vi "external cmd - parse string.vi"(0 "input cmd":string) -> (4 "address":u8, 6 "content":string, 8 "is true":bool, 10 "command ok":bool)   [LabVIEW 2010]
uses:
  <vilib>/Utility/error.llb/whitespace.ctl
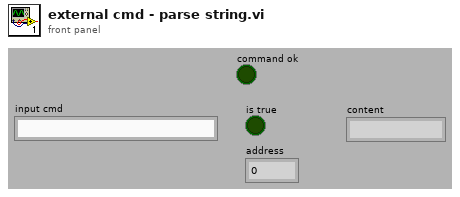
[diagram p1: front panel]
types:
  T1 = typedef "whitespace.ctl" = u16
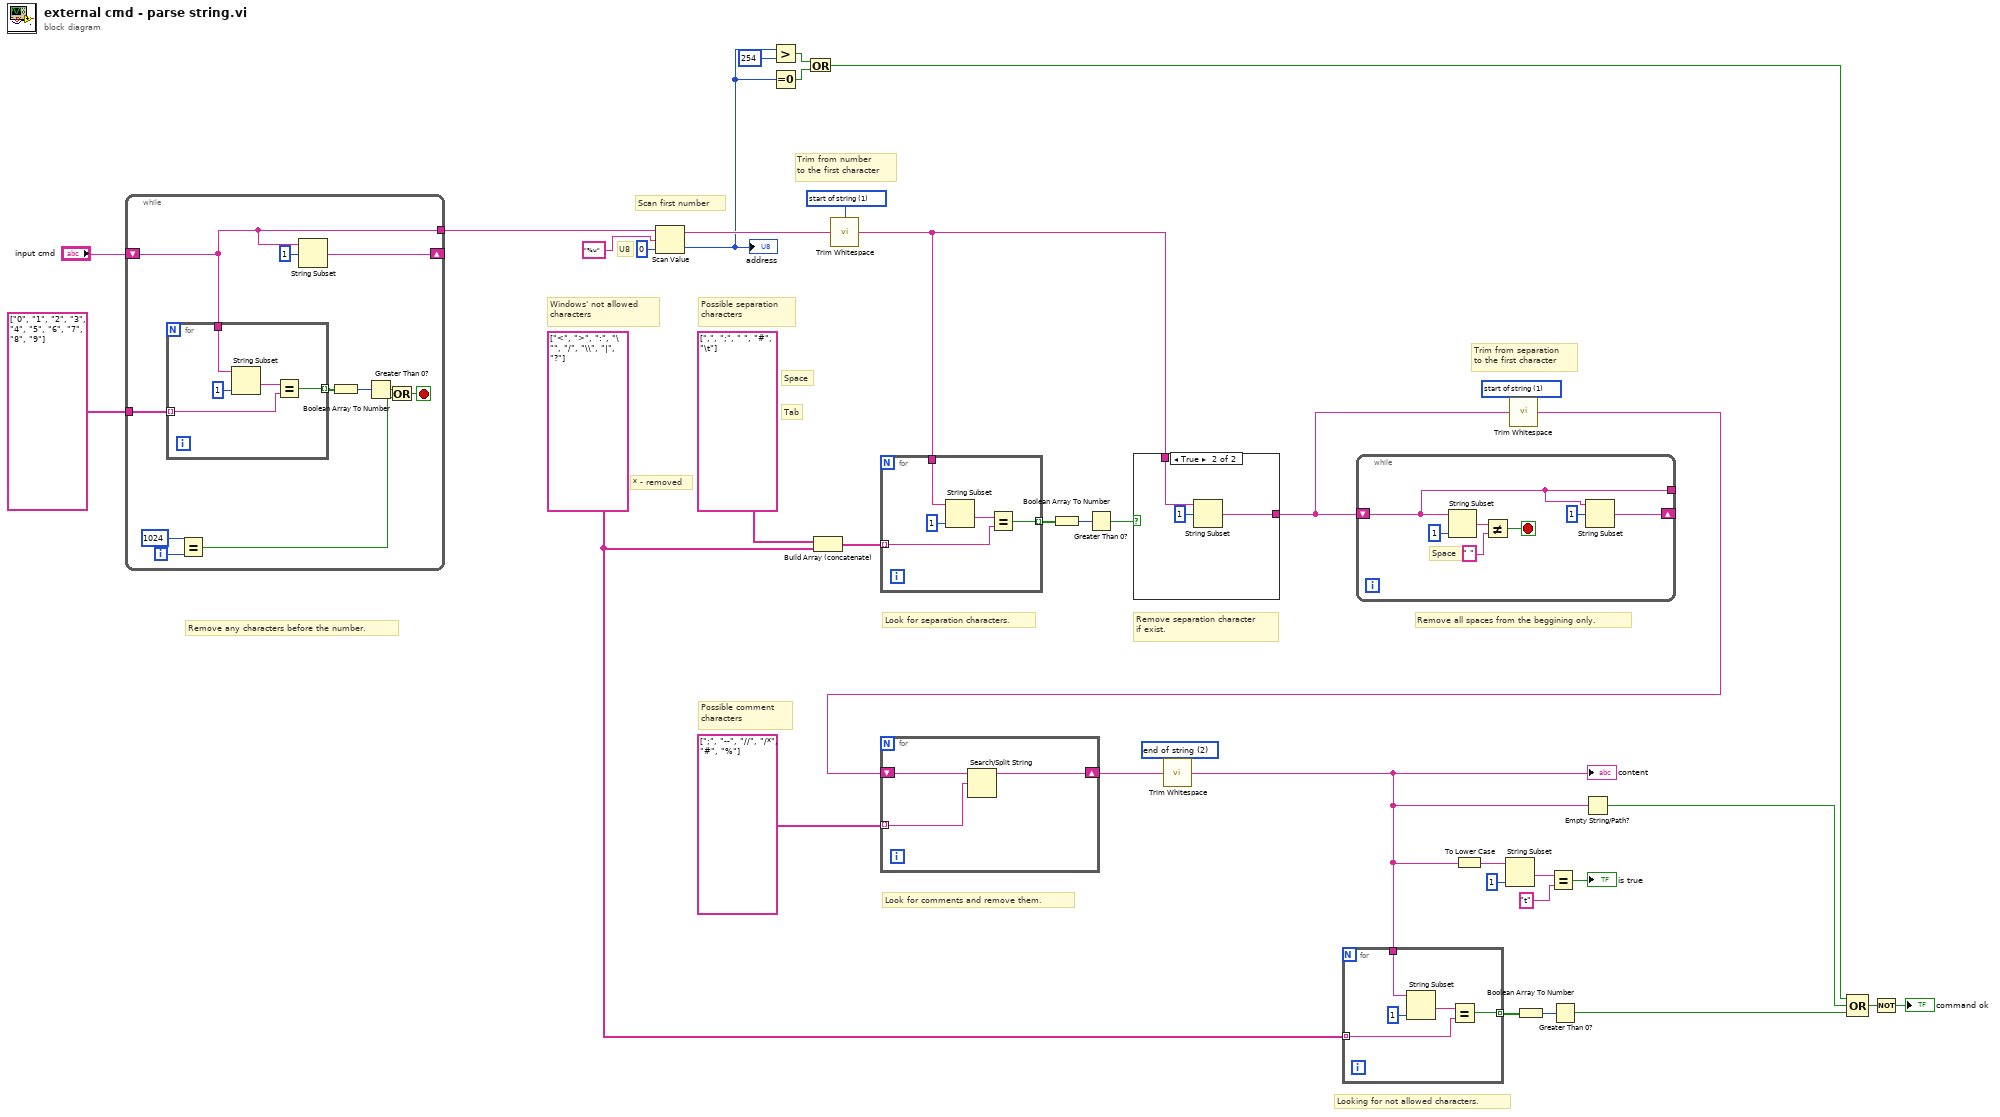
[diagram p0: block diagram]
diagram:
  w19 = T1 1 items=["both", "start of string", "end of string"] ("location (both)")
  w21 = T1 2 items=["both", "start of string", "end of string"] ("location (both)")
  w24 = T1 1 items=["both", "start of string", "end of string"] ("location (both)")
  w18 = string[] ["<", ">", ":", "\"", "/", "\\", "|", "?"]
  # "* - removed"
  # "Looking for not allowed characters."
  # "Trim from separation\nto the first character"
  # "Trim from number\nto the first character"
  # "Scan first number"
  # "Look for comments and remove them."
  # "Possible comment\ncharacters"
  # "Remove all spaces from the beggining only."
  # "Remove separation character\nif exist."
  # "Look for separation characters."
  # "Remove any characters before the number."
  # "Tab"
  # "Space"
  # "U8"
  # "Possible separation\ncharacters"
  # "Windows' not allowed\ncharacters"
  n1 = while {
    shift-right: [w47] -> _
    shift-left: "input cmd" -> [w42]
    tunnel: [w42] -> w28
    tunnel: string[] ["0", "1", "2", "3", "4", "5", "6", "7", "8", "9"] -> [w46]
    i -> [w41]
    stop <- w39 stop-if-true
    n2 = for {
      tunnel: w46 -> [w50] mode=indexing
      tunnel: w42 -> [w53]
      tunnel: [w49] -> w44 mode=indexing
      n3 = String Subset(string=w53, length (rest)=1 ("length (rest)")) -> (substring=w51:string)  [unwired: 1 in]
      n4 = Equal?(x=w51, y=w50) -> (x = y?=w49:bool)
    }
    n5 = Equal?(x=1024, y=w41) -> (x = y?=w38:bool)
    n6 = String Subset(string=w42, offset (0)=1) -> (substring=w47:string)  [unwired: 1 in]
    n7 = Boolean Array To Number(Boolean array=w44) -> (number=w45:u32)
    n8 = Greater Than 0?(x=w45) -> (x > 0?=w43:bool)
    n9 = Or(x=w43, y=w38) -> (x .or. y?=w39:bool)
  }
  n10 = Scan Value(string=w28, format string="%u", default (0 dbl)=u8 0) -> (output string=w25:string, value=w11:u8)
  "address" <- w11
  n11 = Greater?(x=w11, y=u8 254) -> (0:w9:bool)
  n12 = Equal To 0?(x=w11) -> (x = 0?=w10:bool)
  n13 = Or(x=w9, y=w10) -> (x .or. y?=w8:bool)
  n14 = Build Array (concatenate)(string[] [",", ";", " ", "#", "\t"], w18) -> (w35:string[])
  n15 = call <vilib>:"Trim Whitespace.vi"("string"=w25, "location (both)"=w19) -> ("trimmed string"=w20:string)
  n16 = for {
    tunnel: w35 -> [w55] mode=indexing
    tunnel: w20 -> [w58]
    tunnel: [w54] -> w33 mode=indexing
    n17 = String Subset(string=w58, length (rest)=1 ("length (rest)")) -> (substring=w56:string)  [unwired: 1 in]
    n18 = Equal?(x=w56, y=w55) -> (x = y?=w54:bool)
  }
  n19 = Boolean Array To Number(Boolean array=w33) -> (number=w32:u32)
  n20 = Greater Than 0?(x=w32) -> (x > 0?=w31:bool)
  n21 = case shown="True" w31 {
    tunnel: w20 -> [w59 w62]
    tunnel: [w59 w60] -> w23
    frame False {
    }
    frame True {
      n22 = String Subset(string=w62, offset (0)=1) -> (substring=w60:string)  [unwired: 1 in]
    }
  }
  n23 = while {
    shift-right: [w64] -> _
    shift-left: w23 -> [w63]
    tunnel: [w63] -> _
    stop <- w67 stop-if-true
    # "Space"
    n24 = String Subset(string=w63, length (rest)=1 ("length (rest)")) -> (substring=w65:string)  [unwired: 1 in]
    n25 = Not Equal?(x=w65, y=" " ("search string")) -> (x != y?=w67:bool)
    n26 = String Subset(string=w63, offset (0)=1) -> (substring=w64:string)  [unwired: 1 in]
  }
  n27 = call <vilib>:"Trim Whitespace.vi"("string"=w23, "location (both)"=w24) -> ("trimmed string"=w22:string)
  n28 = for {
    tunnel: string[] [";", "--", "//", "/*", "#", "%"] -> [w71] mode=indexing
    shift-right: [w70] -> w26
    shift-left: w22 -> [w72]
    n29 = Search/Split String(string=w72, search string/char (-)=w71) -> (substring before match=w70:string)  [unwired: 1 in, 2 out]
  }
  n30 = call <vilib>:"Trim Whitespace.vi"("string"=w26, "location (both)"=w21) -> ("trimmed string"=w14:string)
  "content" <- w14
  n31 = for {
    tunnel: w18 -> [w74] mode=indexing
    tunnel: w14 -> [w77]
    tunnel: [w73] -> w16 mode=indexing
    n32 = String Subset(string=w77, length (rest)=1 ("length (rest)")) -> (substring=w75:string)  [unwired: 1 in]
    n33 = Equal?(x=w75, y=w74) -> (x = y?=w73:bool)
  }
  n34 = To Lower Case(string=w14) -> (all lower case string=w5:string)
  n35 = String Subset(string=w5, length (rest)=1 ("length (rest)")) -> (substring=w7:string)  [unwired: 1 in]
  n36 = Boolean Array To Number(Boolean array=w16) -> (number=w17:u32)
  n37 = Equal?(x=w7, y="t" ("search string")) -> (x = y?=→"is true":bool)
  n38 = Greater Than 0?(x=w17) -> (x > 0?=w15:bool)
  n39 = Empty String/Path?(string/path=w14) -> (empty?=w13:bool)
  n40 = Compound Arithmetic op=OR(w8, w13, w15) -> (w2:bool)
  n41 = Not(x=w2) -> (.not. x?=→"command ok":bool)
